vi "echo.vi"() -> (0 "error out":errorcluster)   [LabVIEW 2014, in "lv-build-library.lvlib"]
uses:
  lv-build-library.lvlib
  <vilib>/Wiresmith Technology/LabVIEW CLI/CLI Class/CLI.lvclass
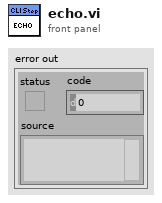
[diagram p1: front panel]
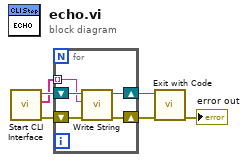
[diagram p0: block diagram]
diagram:
  n1 = call <vilib>:"Start CLI Interface.vi"() -> ("error out"=w4:errorcluster, "Custom Parameters"=w5:string[], "CLI out"=w6:refnum<class "CLI.lvclass">)  [unwired: 9 in]
  n2 = for {
    shift-right: [w7] -> w3
    shift-left: w6 -> [w11]
    tunnel: w5 -> [w10] mode=indexing
    shift-right: [w8] -> w2
    shift-left: w4 -> [w9]
    n3 = call <vilib>:"Write String.vi"("error in (no error)"=w9, "Text to Write"=w10, "CLI in"=w11) -> ("error out"=w8:errorcluster, "CLI out"=w7:refnum<class "CLI.lvclass">)  [unwired: 7 in]
  }
  n4 = call <vilib>:"Exit with Code.vi"("error in (no error)"=w2, "CLI in"=w3) -> ("error out"=→"error out":errorcluster)  [unwired: 9 in]
